vi "Ball Vomit.vi"(8 "Rear Roller Speed":dbl, 9 "Front Roller Speed":dbl, 10 "Roller Time":u32, 11 "Wait Time(ms)":u32) -> ()   [LabVIEW 2011]
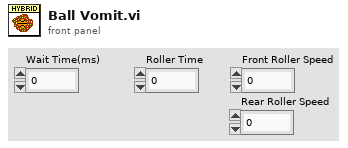
[diagram p1: front panel]
types:
  T1 = typedef "WPI_MotorControlDeviceRef.ctl" = cluster{"DeviceStatus":errorcluster, "Type":enum16{"PWM", "CAN"}, "PWM":cluster{"Digital Module":T2, "PWM Channel":T3, "DeadBand":T4}, "CAN":cluster{"Device Number":u8, "Control Mode":T5, "Semaphore":T6, "Max Vout":dbl}, "Invert":bool, "TransformRef":T7, "InvTransformRef":T7}
  T2 = typedef "FPGA_TypedefDigitalModule.ctl" = enum16{"Digital Module 1", "Digital Module 2"}
  T3 = typedef "FPGA_DIOPWMChannel.ctl" = enum8{"PWM 1", "PWM 2", "PWM 3", "PWM 4", "PWM 5", "PWM 6", "PWM 7", "PWM 8", "PWM 9", "PWM 10", "Invalid"}
  T4 = typedef "WPI_PWMDeadband.ctl" = cluster{"Name":string, "maxPositivePwm":i32, "minPositivePwm":i32, "centerPwm":i32, "maxNegativePwm":i32, "minNegativePwm":i32, "angularRange":u16}
  T5 = typedef "WPI_CANJaguar_ControlMode.ctl" = enum8{"Percent VBus", "Current", "Speed", "Position", "Voltage"}
  T6 = typedef "Semaphore RefNum" = refnum<k1>
  T7 = typedef "WPI_PWMTransform_ConPane.ctl" = refnum<vi>
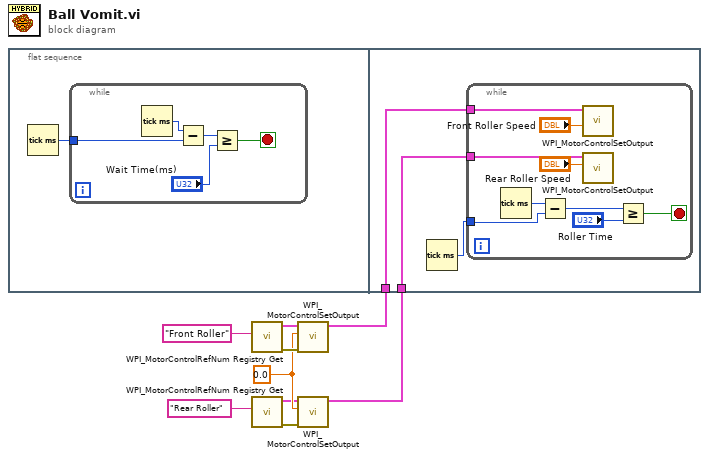
[diagram p0: block diagram]
diagram:
  w5 = 0.0 ("RelayValue")
  n1 = flat-sequence {
    tunnel: w4 -> [w16]
    tunnel: w3 -> [w17]
    frame #0 {
      n2 = Tick Count (ms)() -> (millisecond timer value=w10:u32)
      n3 = while {
        tunnel: w10 -> [w14]
        stop <- w11 stop-if-true
        n4 = Tick Count (ms)() -> (millisecond timer value=w15:u32)
        n5 = Subtract(x=w15, y=w14) -> (x-y=w13:u32)
        n6 = Greater Or Equal?(x=w13, y="Wait Time(ms)") -> (x >= y?=w11:bool)
      }
    }
    frame #1 {
      n7 = Tick Count (ms)() -> (millisecond timer value=w18:u32)
      n8 = while {
        tunnel: w18 -> [w24]
        tunnel: w17 -> [w22]
        tunnel: w16 -> [w21]
        stop <- w25 stop-if-true
        n9 = Tick Count (ms)() -> (millisecond timer value=w27:u32)
        n10 = Subtract(x=w27, y=w24) -> (x-y=w26:u32)
        n11 = call <vilib>:"WPI_MotorControlSetOutput.vi"("Output"="Front Roller Speed", "MotorControlDevRef"=w22) -> ()  [unwired: 8 in, 2 out]
        n12 = call <vilib>:"WPI_MotorControlSetOutput.vi"("Output"="Rear Roller Speed", "MotorControlDevRef"=w21) -> ()  [unwired: 8 in, 2 out]
        n13 = Greater Or Equal?(x=w26, y="Roller Time") -> (x >= y?=w25:bool)
      }
    }
  }
  n14 = call <vilib>:"WPI_MotorControlRefNum Registry Get.vi"("refnum name"="Front Roller") -> ("error out"=w7:errorcluster, "MotorControlDevRef"=w2:T1)  [unwired: 9 in]
  n15 = call <vilib>:"WPI_MotorControlRefNum Registry Get.vi"("refnum name"="Rear Roller") -> ("error out"=w6:errorcluster, "MotorControlDevRef"=w1:T1)  [unwired: 9 in]
  n16 = call <vilib>:"WPI_MotorControlSetOutput.vi"("error in (no error)"=w7, "Output"=w5, "MotorControlDevRef"=w2) -> ("MotorControlDevRef"=w3:T1)  [unwired: 7 in, 1 out]
  n17 = call <vilib>:"WPI_MotorControlSetOutput.vi"("error in (no error)"=w6, "Output"=w5, "MotorControlDevRef"=w1) -> ("MotorControlDevRef"=w4:T1)  [unwired: 7 in, 1 out]
